vi "Initialize Devices (SubVI).vi"(11 "deviceKey":string) -> (0 "sortie d'erreur":errorcluster, 1 "DeviceKey List Out":string[](array[string]), 2 "Device Array":T1(array[cluster]), 3 "Refnum de .NET en sortie":refnum<k24>)   [LabVIEW 2017]
doc: "by Tanguy BOULARD"
uses:
  dll/CmdLib.dll
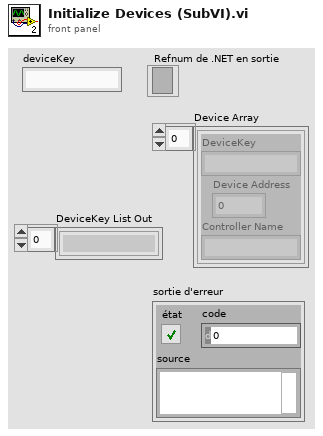
[diagram p1: front panel]
types:
  T1 = cluster{"DeviceKey":string, "Device Address":i32, "Controller Name":string}[]
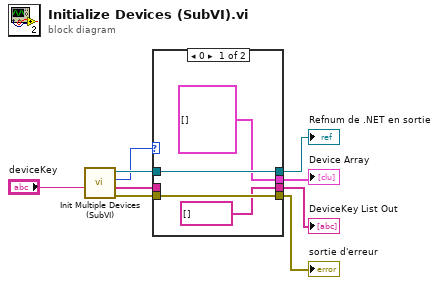
[diagram p0: block diagram]
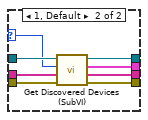
[diagram p2: hidden frame]
diagram:
  n1 = call "Init Multiple Devices (SubVI).vi"("deviceKey"="deviceKey") -> ("sortie d'erreur"=w3:errorcluster, "GetDeviceKeys"=w5:string[], "Numérique"=w2:i32, "Refnum de .NET en sortie"=w4:refnum<k24>)  [unwired: 7 in]
  n2 = case shown="0" w2 {
    selector: w2 -> [_ w18]
    tunnel: w3 -> [w12 w21]
    tunnel: w4 -> [w13 w19]
    tunnel: w5 -> [_ w20]
    tunnel: [w12 w17] -> w8
    tunnel: [T1 [] ("Device Array") w16] -> w7
    tunnel: [w13 w15] -> w6
    tunnel: [string[] [] ("DeviceKey List Out") w14] -> w1
    frame 0 {
    }
    frame 1, Default {
      n3 = call "Get Discovered Devices (SubVI).vi"("error in"=w21, "DeviceKey List"=w20, "Master Count"=w18, "CmdLib In"=w19) -> ("error out"=w17:errorcluster, "DeviceKey List Out"=w14:string[], "Device Array"=w16:T1, "CmdLib Out"=w15:refnum<k24>)  [unwired: 4 in]
    }
  }
  "Refnum de .NET en sortie" <- w6
  "Device Array" <- w7
  "sortie d'erreur" <- w8
  "DeviceKey List Out" <- w1
